vi "Open.vi"(7 "Config data in":variant, 8 "error in (no error)":errorcluster, 9 "Timeout (ms)":u32=3000, 10 "VISA session":refnum<visa-resource-name>="TCPIP::146.201.232.88::7180::SOCKET", 11 "PS Driver.lvlib:PS Driver.lvclass in":refnum<class "PS Driver.lvclass">) -> (0 "error out":errorcluster, 1 "Config data out":variant, 2 "dup VISA Session":refnum<visa-resource-name>, 3 "PS Driver.lvlib:PS Driver.lvclass out":refnum<class "PS Driver.lvclass">)   [LabVIEW 2025, in "PS Driver.lvlib" / "PS Driver.lvclass"]
doc: "Author: Scott Hannahs <sth@magnet.fsu.edu>\n\nThis software is licensed for use under the “MIT License\"\nCopyright (c) 2025 Scott Hannahs, sth@sth@magnet.sthnet.net\n\nPermission is hereby granted, free of charge, to any person obtaining a copy of this software and associated documentation files (the \"Software\"), to deal in the Software without restriction, including without limitation the rights to use, copy, modify, merge, publish, distribute, sublicense, and/or sell copies of the Software, and to permit persons to whom the Software is furnished to do so, subject to the following conditions: The above copyright notice and this permission notice shall be included in all copies or substantial portions of the Software.\n\nTHE SOFTWARE IS PROVIDED \"AS IS\", WITHOUT WARRANTY OF ANY KIND, EXPRESS OR IMPLIED, INCLUDING BUT NOT LIMITED TO THE WARRANTIES OF MERCHANTABILITY, FITNESS FOR A PARTICULAR PURPOSE AND NONINFRINGEMENT. IN NO EVENT SHALL THE AUTHORS OR COPYRIGHT HOLDERS BE LIABLE FOR ANY CLAIM, DAMAGES OR OTHER LIABILITY, WHETHER IN AN ACTION OF CONTRACT, TORT OR OTHERWISE, ARISING FROM, OUT OF OR IN CONNECTION WITH THE SOFTWARE OR THE USE OR OTHER DEALINGS IN THE SOFTWARE."
uses:
  PS Driver.lvclass
  PS Driver.lvclass/PS Driver.ctl
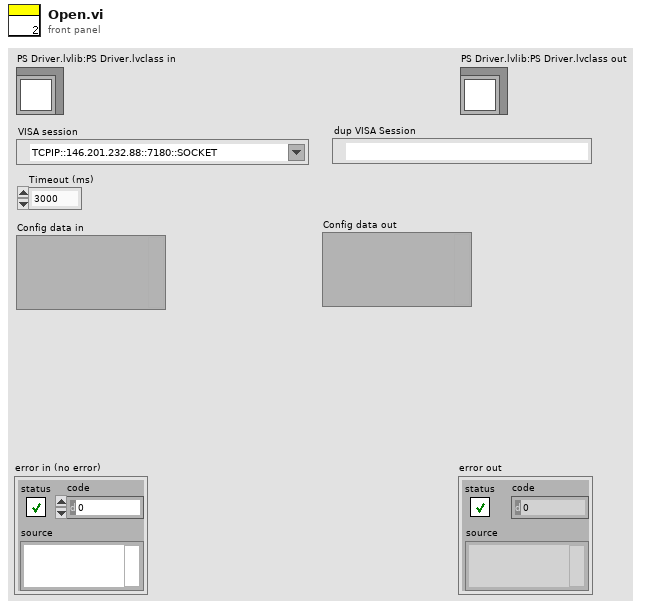
[diagram p1: front panel]
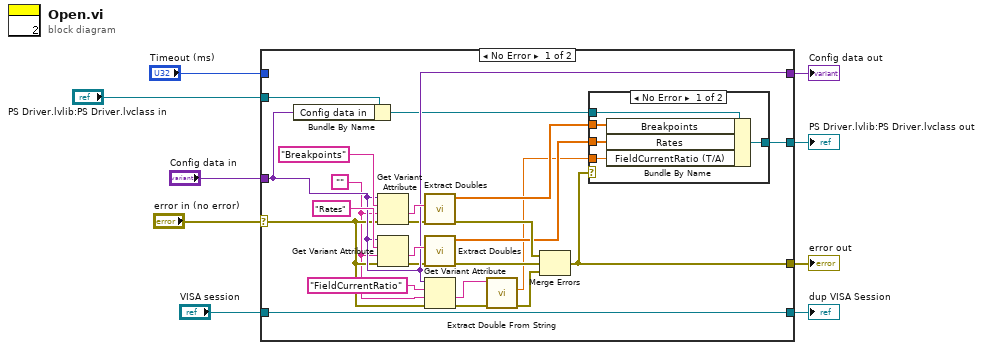
[diagram p0: block diagram]
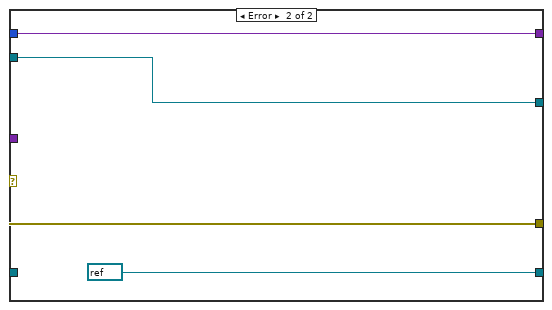
[diagram p3: hidden frame]
diagram:
  n1 = case shown="No Error" "error in (no error)" {
    selector: "error in (no error)" -> [w25 w42]
    tunnel: [w18 w42] -> w8
    tunnel: [w14 w41] -> w6
    tunnel: "PS Driver.lvlib:PS Driver.lvclass in" -> [w32 w41]
    tunnel: "VISA session" -> [w23 _]
    tunnel: "Timeout (ms)" -> [_ _]
    tunnel: "Config data in" -> [w26 w39]
    tunnel: [w23 refnum<visa-resource-name> refnum ("dup VISA Session")] -> w2
    tunnel: [w26 w39] -> w1
    frame No Error {
      w24 = ""
      n2 = Bundle By Name(cluster=w32, "Config data in"=w26) -> (w17:refnum<class "PS Driver.lvclass">)
      n3 = Get Variant Attribute(Variant=w26, name="Breakpoints", default value (empty Variant)=w24, error in=w25) -> (value=w29:string, error out=w22:errorcluster)  [unwired: 2 out]
      n4 = Get Variant Attribute(Variant=w26, name="Rates", default value (empty Variant)=w24, error in=w25) -> (value=w28:string, error out=w20:errorcluster)  [unwired: 2 out]
      n5 = call "Extract Doubles.vi"("error in"=w22, "String"=w29) -> ("error out"=w21:errorcluster, "Data"=w16:dbl[])  [unwired: 4 in]
      n6 = call "Extract Doubles.vi"("error in"=w20, "String"=w28) -> ("error out"=w19:errorcluster, "Data"=w15:dbl[])  [unwired: 4 in]
      n7 = Get Variant Attribute(Variant=w26, name="FieldCurrentRatio", default value (empty Variant)=w24, error in=w25) -> (value=w13:string, error out=w12:errorcluster)  [unwired: 2 out]
      n8 = call "Extract Double From String.vi"("error in"=w12, "string"=w13) -> ("error out"=w11:errorcluster, "floating pt. number"=w10:dbl)  [unwired: 2 in, 2 out]
      n9 = Merge Errors(w21, w19, w11) -> (w18:errorcluster)
      n10 = case shown="No Error" w18 {
        tunnel: w17 -> [w37 w38]
        tunnel: w16 -> [w36 _]
        tunnel: w15 -> [w35 _]
        tunnel: w10 -> [w34 _]
        tunnel: [w33 w38] -> w14
        frame No Error {
          n11 = Bundle By Name(cluster=w37, "Breakpoints"=w36, "Rates"=w35, "FieldCurrentRatio (T/A)"=w34) -> (w33:refnum<class "PS Driver.lvclass">)
        }
        frame Error {
        }
      }
    }
    frame Error {
    }
  }
  "error out" <- w8
  "PS Driver.lvlib:PS Driver.lvclass out" <- w6
  "dup VISA Session" <- w2
  "Config data out" <- w1
